vi "Read Samples.vi"(0 "Filename":path, 5 "channel":i32, 7 "offset in":i32, 9 "Npts":i32, 11 "error in (no error)":errorcluster) -> (4 "Samples":dbl[](array[numeric]), 8 "offset out":i32, 10 "end of file?":bool, 15 "error out":errorcluster)   [LabVIEW 2020, in "File.lvclass"]
uses:
  File.lvclass
  <vilib>/sound2/lvsound2.llb/Sound File Position.ctl
  <vilib>/sound2/lvsound2.llb/Sound File Read Open.vi
  <vilib>/sound2/lvsound2.llb/Sound File Read (DBL).vi
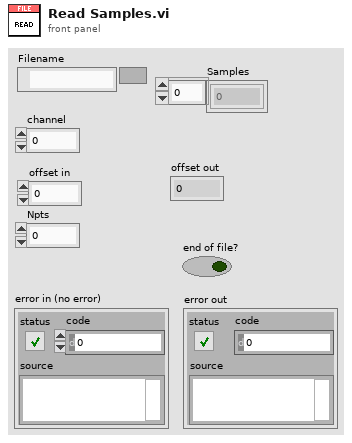
[diagram p1: front panel]
types:
  T1 = enum16{"open", "replace", "create", "open or create", "replace or create", "replace or create with confirmation"}
  T2 = typedef "Sound File Position.ctl" = u16
  T3 = typedef "Sound File Refnum.ctl" = refnum<file>
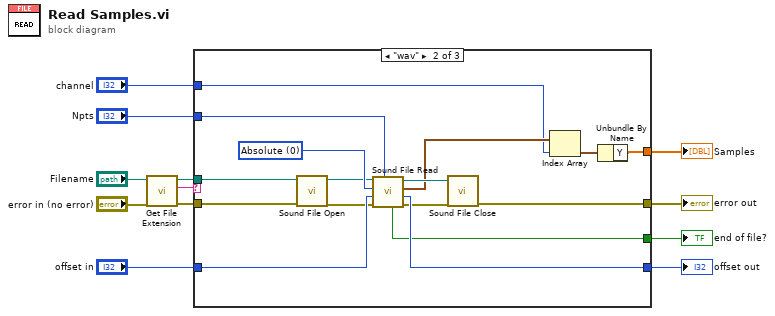
[diagram p0: block diagram]
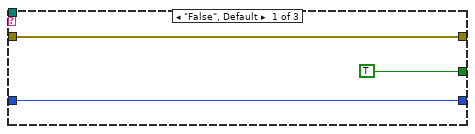
[diagram p2: hidden frame]
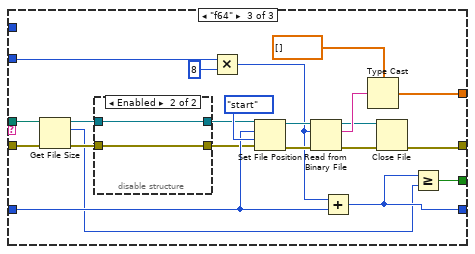
[diagram p3: hidden frame]
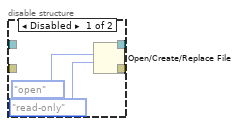
[diagram p4: hidden frame]
diagram:
  n1 = call <vilib>:"Get File Extension.vi"("error in (no error)"="error in (no error)", "file"="Filename") -> ("error out"=w3:errorcluster, "lowercase file extension"=w1:string, "dup file"=w2:path)  [unwired: 5 in, 2 out]
  n2 = case shown="\"wav\"" w1 {
    tunnel: [w15 w31 w33] -> w12
    tunnel: [TRUE ("end of file?") w30 w34] -> w11
    tunnel: "offset in" -> [w15 w29 w42]
    tunnel: "Npts" -> [_ w27 w50]
    tunnel: [w14 w26 w43] -> w8
    tunnel: "channel" -> [_ w19 _]
    tunnel: [_ w18 w46] -> w6
    tunnel: w3 -> [w14 w17 w40]
    tunnel: w2 -> [_ w16 w39]
    frame "False", Default {
    }
    frame "wav" {
      w28 = T2 0 items=["Absolute"=0, "Relative"=2] ("position mode")
      n3 = call-poly <vilib>:"Sound File Open.vi"("error in (no error)"=w17, "path"=w16) -> ("error out"=w23:errorcluster, "sound file refnum"=w22:T3)  [unwired: 8 in]
      n4 = call-poly <vilib>:"Sound File Read.vi"("number of samples/ch (-1: all)"=w27, "error in (no error)"=w23, "position offset"=w29, "position mode"=w28, "sound file refnum"=w22) -> ("error out"=w24:errorcluster, "offset"=w31:i32, "data"=w20:waveform(dbl)[], "sound file refnum out"=w25:T3, "end of file?"=w30:bool)  [unwired: 2 in]
      n5 = call <vilib>:"Sound File Close.vi"("error in (no error)"=w24, "sound file refnum"=w25) -> ("error out"=w26:errorcluster)  [unwired: 9 in]
      n6 = Index Array(array=w20, index=w19) -> (element=w21:waveform(dbl))
      n7 = Unbundle By Name(w21) -> ("Y"=w18:dbl[])
    }
    frame "f64" {
      n8 = Get File Size(file=w39, error in=w40) -> (refnum out=w38:refnum<file>, size (in bytes)=w32:i64, 0:w36:errorcluster)
      n9 = disable-structure shown="Enabled" {
        disable-tunnel: w38 -> [_ w57]
        disable-tunnel: [_ w57] -> w37
        disable-tunnel: w36 -> [_ w56]
        disable-tunnel: [_ w56] -> w35
        frame Disabled {
          n10 = Open/Create/Replace File(operation (0:open)=T1."open", access (0:read/write)=enum16{"read/write", "read-only", "write-only"}."read-only") -> ()  [unwired: 4 in, 3 out]
        }
        frame Enabled {
        }
      }
      n11 = Multiply(x=w50, y=8) -> (x*y=w41:i32)
      n12 = Set File Position(offset (in bytes) (0)=w42, refnum=w37, from (0:start)=enum16{"start", "end", "current"}."start", error in=w35) -> (refnum out=w51:refnum<file>, error out=w52:errorcluster)
      n13 = Read from Binary File(8:w52, 10:w41, 11:w51) -> (0:w44:errorcluster, 2:w48:string, 3:w45:refnum<file>)  [unwired: 3 in, 1 out]
      n14 = Add(x=w41, y=w42) -> (x+y=w33:i32)
      n15 = Type Cast(type=dbl[] [] ("Y"), x=w48) -> (*(type *) &x=w46:dbl[])
      n16 = Close File(refnum=w45, error in=w44) -> (error out=w43:errorcluster)  [unwired: 1 out]
      n17 = Greater Or Equal?(x=w33, y=w32) -> (x >= y?=w34:bool)
    }
  }
  "offset out" <- w12
  "end of file?" <- w11
  "error out" <- w8
  "Samples" <- w6
